vi "InstrParams.vi"() -> ()   [LabVIEW 2014, in "GenericDAQ.lvlib"]
uses:
  <instrlib>/GenericDAQ/GenericDAQ.lvlib
panel:
  in  "Instr.Params":dbl[](array[numeric])
  in  "TriggerRate":u32=1000
  in  "SignalOn":bool=TRUE
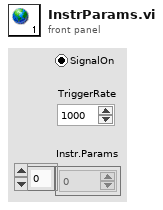
[diagram p1: front panel]
diagram:
